vi "Main.vi"() -> ()   [LabVIEW 2018]
uses:
  Data Def/Com Port.ctl
  Data Def/Device.ctl
  <userlib>/_MGI/Timing/MGI Wait/MGI Wait (U32).vi
panel:
  in  "KFM Disconnect PLZ":bool
  in  "KFM Connect PLZ":bool
  in  "Stop Load":bool
  in  "Apply Load":bool
  out "Com Port":T1
  out "Run Count":i32
  out "Setting Tab":T2(tab)
  in  "Apply PLZ Setting":bool
  in  "Operation Mode":u16(ring) items=["Constant Current(CC)", "Constant Voltage(CV)", "Constant Power(CP)", "Constant Resistance(CR)", "Constant Current & Voltage(CCCV)", "Constant Resistance & Voltage(CRCV)"]
  out "Error":errorcluster
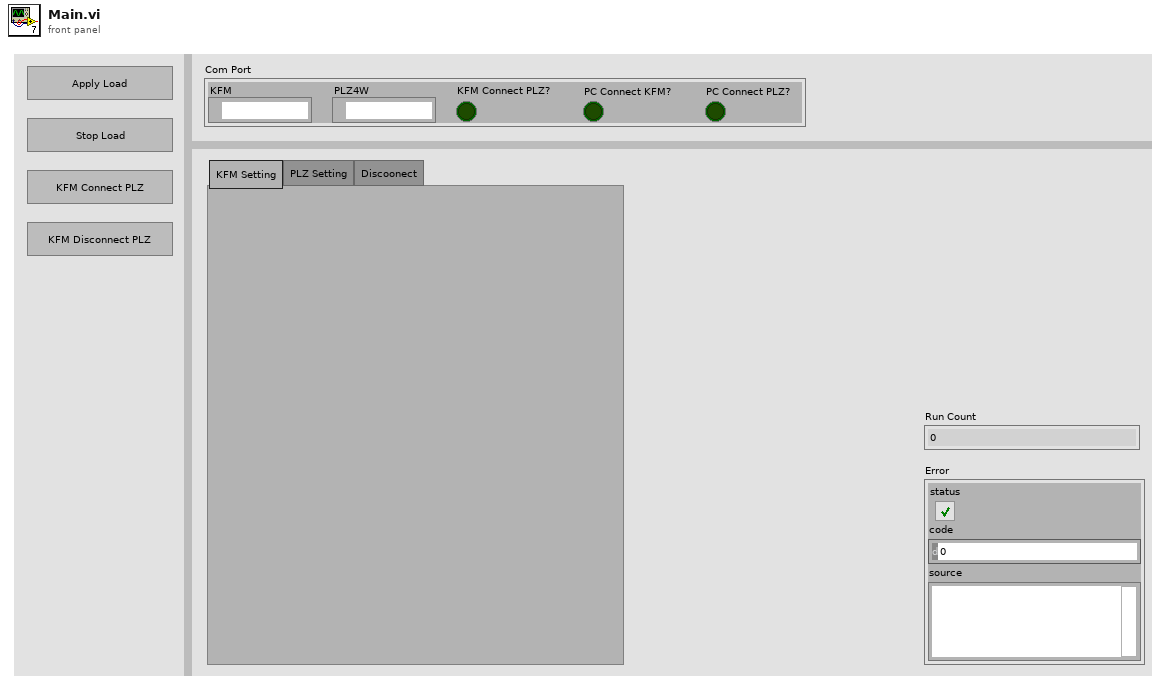
[diagram p1: front panel]
types:
  T1 = typedef "Com Port.ctl" = cluster{"KFM":refnum<visa-resource-name>, "PLZ4W":refnum<visa-resource-name>, "KFM Connect PLZ?":bool, "PC Connect KFM?":bool, "PC Connect PLZ?":bool}
  T2 = enum32{"KFM Setting", "PLZ Setting", "Discoonect"}
  T3 = typedef "Device.ctl" = enum16{"KFM", "PLZ"}
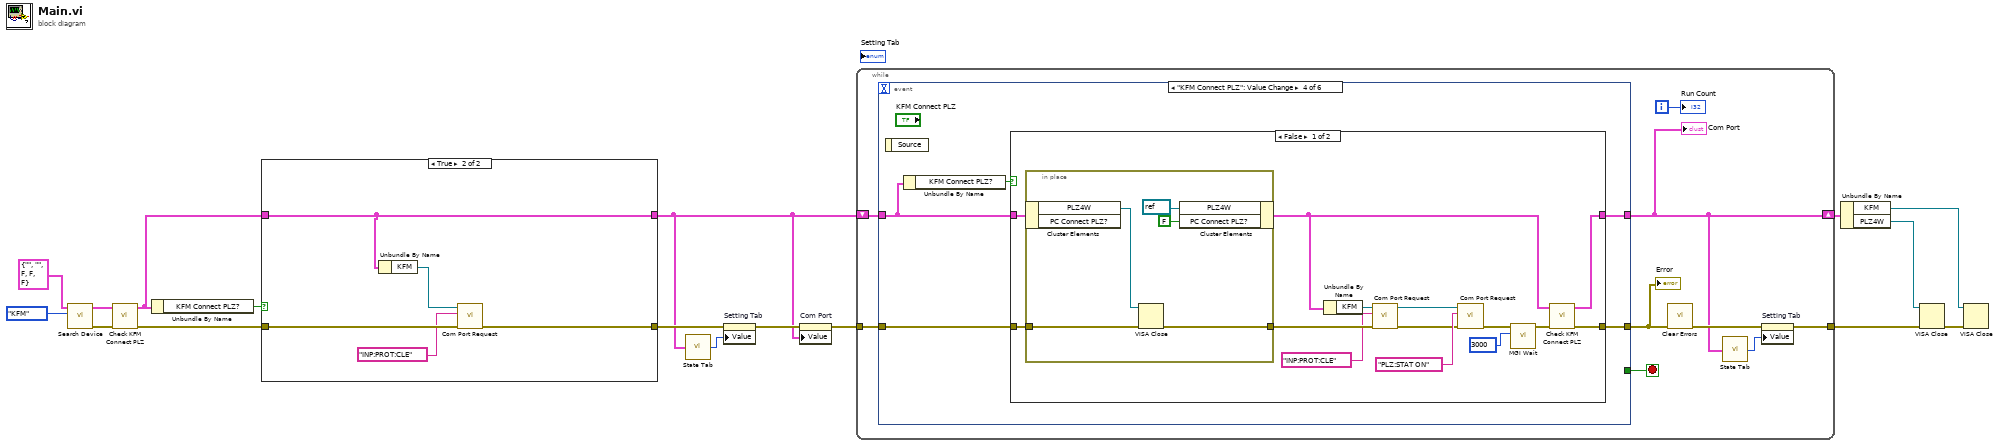
[diagram p0: block diagram]
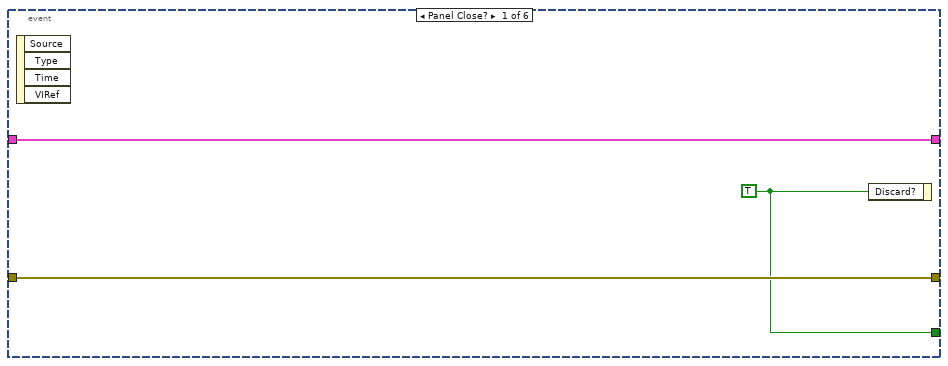
[diagram p2: hidden frame]
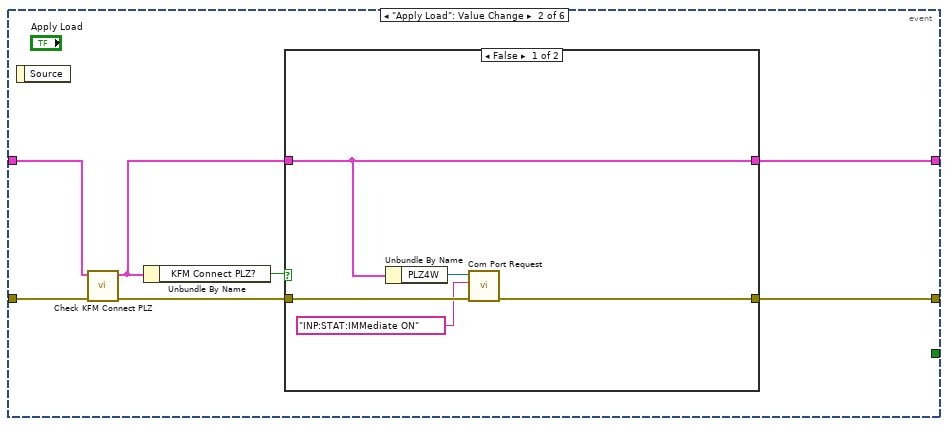
[diagram p3: hidden frame]
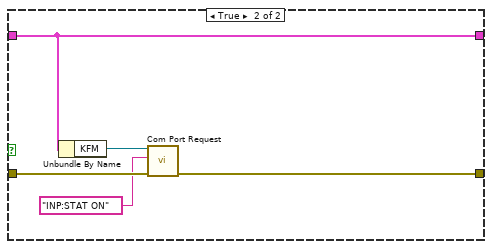
[diagram p4: hidden frame]
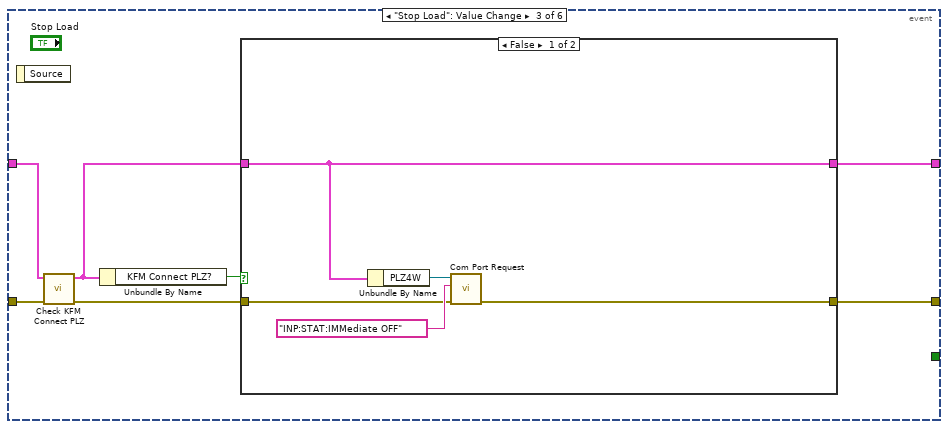
[diagram p5: hidden frame]
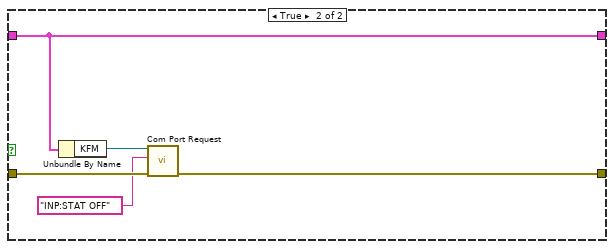
[diagram p6: hidden frame]
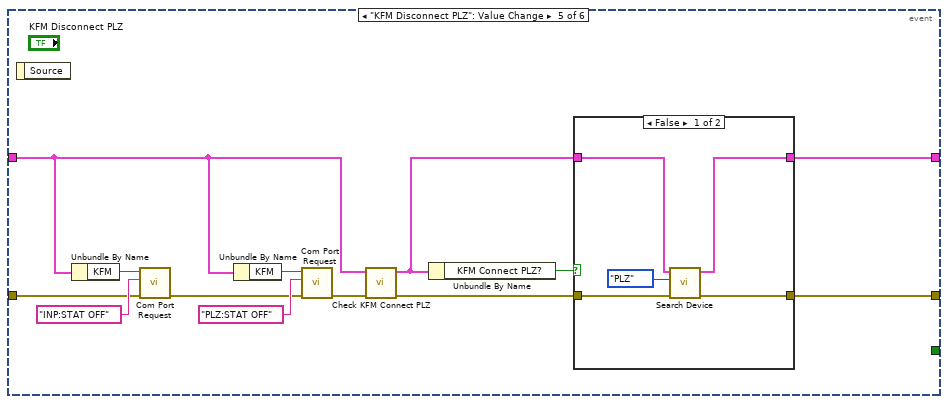
[diagram p8: hidden frame]
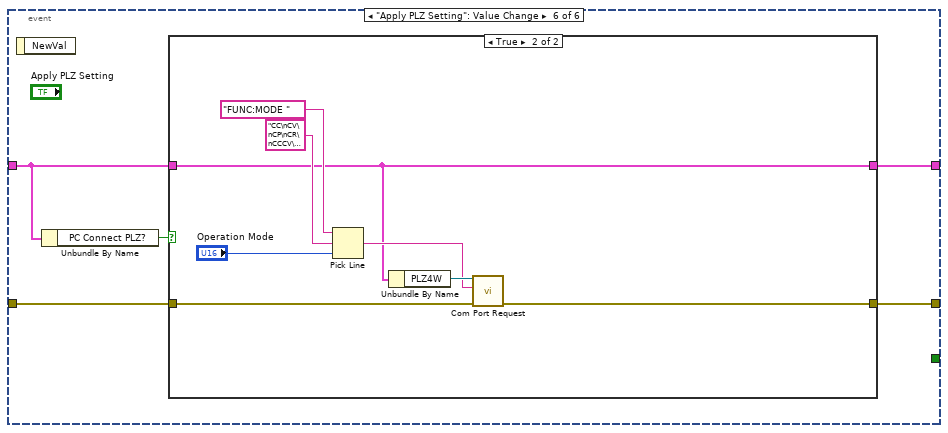
[diagram p10: hidden frame]
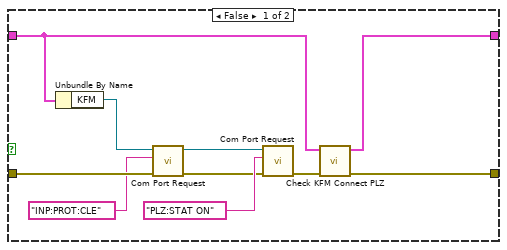
[diagram p12: hidden frame]
diagram:
  n1 = call "Search Device.vi"("Device"=Device."KFM", "Com Port In"=T1 {"KFM"="", "PLZ4W"="", "KFM Connect PLZ?"=FALSE, "PC Connect KFM?"=FALSE, "PC Connect PLZ?"=FALSE} ("Com Port")) -> ("error out"=w11:errorcluster, "Com Port Out"=w10:T1)  [unwired: 8 in]
  n2 = call "Check KFM Connect PLZ.vi"("error in"=w11, "Com Port In"=w10) -> ("error out"=w13:errorcluster, "Com Port Out"=w6:T1)  [unwired: 8 in]
  n3 = Unbundle By Name(w6) -> ("KFM Connect PLZ?"=w7:bool)
  n4 = case shown="True" w7 {
    tunnel: w13 -> [w19 w31]
    tunnel: w6 -> [w25 w29]
    tunnel: [w23 w29] -> w2
    tunnel: [w24 w28] -> w5
    frame False {
      n5 = Unbundle By Name(w25) -> ("KFM"=w21:refnum<visa-resource-name>)
      n6 = call "Com Port Request.vi"("error in"=w19, "Command"="INP:PROT:CLE", "Com Port In"=w21) -> ("error out"=w22:errorcluster, "Com Port Out"=w20:refnum<visa-resource-name>)  [unwired: 6 in, 1 out]
      n7 = call "Com Port Request.vi"("error in"=w22, "Command"="PLZ:STAT ON", "Com Port In"=w20) -> ("error out"=w26:errorcluster)  [unwired: 6 in, 2 out]
      n8 = call "Check KFM Connect PLZ.vi"("error in"=w26, "Com Port In"=w25) -> ("error out"=w24:errorcluster, "Com Port Out"=w23:T1)  [unwired: 8 in]
    }
    frame True {
      n9 = Unbundle By Name(w29) -> ("KFM"=w32:refnum<visa-resource-name>)
      n10 = call "Com Port Request.vi"("error in"=w31, "Command"="INP:PROT:CLE", "Com Port In"=w32) -> ("error out"=w28:errorcluster)  [unwired: 6 in, 2 out]
    }
  }
  n11 = call "State Tab.vi"("Com Port"=w2) -> ("Setting Tab"=w4:T2)
  n12 = property on="Setting Tab" class="TabCtl (strict)"(error in=w5, "Value"=w4) -> (error out=w3:errorcluster)  [unwired: 1 in, 1 out]
  n13 = property on="Com Port" class="Clust (strict)"(error in=w3, "Value"=w2) -> (error out=w1:errorcluster)  [unwired: 1 in, 1 out]
  n14 = while {
    tunnel: w1 -> [w40]
    shift-right: [w33] -> w14
    shift-left: w2 -> [w41]
    tunnel: [w34] -> w12
    i -> [w37]
    stop <- w39 stop-if-true
    n15 = event shown="[3] \"KFM Connect PLZ\": Value Change" {
      selector: _ -> [_ _ _ _ _ _]
      dyn-events: _ -> [_ _ _ _ _ _]
      timeout: _ -> [_ _ _ _ _ _]
      tunnel: w41 -> [w44 w47 w66 w80 w105 w128]
      tunnel: w40 -> [w43 w48 w68 w83 w107 w127]
      tunnel: [w44 w46 w64 w82 w113 w125] -> w33
      tunnel: [w43 w45 w65 w81 w114 w126] -> w38
      tunnel: [w42 _ _ _ _ _] -> w39
      event Panel Close? {
        w42 = TRUE ("Discard?")
        n16 = event-data() -> ()  [unwired: 1 in, 4 out]
        n17 = event-data("Discard?"=w42) -> ()  [unwired: 1 in, 1 out]
      }
      event "Apply Load": Value Change {
        n18 = event-data() -> ()  [unwired: 1 in, 1 out]
        n19 = call "Check KFM Connect PLZ.vi"("error in"=w48, "Com Port In"=w47) -> ("error out"=w51:errorcluster, "Com Port Out"=w50:T1)  [unwired: 8 in]
        n20 = Unbundle By Name(w50) -> ("KFM Connect PLZ?"=w49:bool)
        n21 = case shown="False" w49 {
          tunnel: w51 -> [w56 w61]
          tunnel: w50 -> [w52 w58]
          tunnel: [w53 w59] -> w45
          tunnel: [w52 w58] -> w46
          frame False {
            n22 = Unbundle By Name(w52) -> ("PLZ4W"=w55:refnum<visa-resource-name>)
            n23 = call "Com Port Request.vi"("error in"=w56, "Command"="INP:STAT:IMMediate ON", "Com Port In"=w55) -> ("error out"=w53:errorcluster)  [unwired: 6 in, 2 out]
          }
          frame True {
            n24 = Unbundle By Name(w58) -> ("KFM"=w60:refnum<visa-resource-name>)
            n25 = call "Com Port Request.vi"("error in"=w61, "Command"="INP:STAT ON", "Com Port In"=w60) -> ("error out"=w59:errorcluster)  [unwired: 6 in, 2 out]
          }
        }
      }
      event "Stop Load": Value Change {
        n26 = event-data() -> ()  [unwired: 1 in, 1 out]
        n27 = call "Check KFM Connect PLZ.vi"("error in"=w68, "Com Port In"=w66) -> ("error out"=w67:errorcluster, "Com Port Out"=w63:T1)  [unwired: 8 in]
        n28 = Unbundle By Name(w63) -> ("KFM Connect PLZ?"=w62:bool)
        n29 = case shown="False" w62 {
          tunnel: w67 -> [w71 w78]
          tunnel: w63 -> [w70 w75]
          tunnel: [w69 w76] -> w65
          tunnel: [w70 w75] -> w64
          frame False {
            n30 = Unbundle By Name(w70) -> ("PLZ4W"=w73:refnum<visa-resource-name>)
            n31 = call "Com Port Request.vi"("error in"=w71, "Command"="INP:STAT:IMMediate OFF", "Com Port In"=w73) -> ("error out"=w69:errorcluster)  [unwired: 6 in, 2 out]
          }
          frame True {
            n32 = Unbundle By Name(w75) -> ("KFM"=w77:refnum<visa-resource-name>)
            n33 = call "Com Port Request.vi"("error in"=w78, "Command"="INP:STAT OFF", "Com Port In"=w77) -> ("error out"=w76:errorcluster)  [unwired: 6 in, 2 out]
          }
        }
      }
      event "KFM Connect PLZ": Value Change {
        n34 = event-data() -> ()  [unwired: 1 in, 1 out]
        n35 = Unbundle By Name(w80) -> ("KFM Connect PLZ?"=w79:bool)
        n36 = case shown="False" w79 {
          tunnel: w83 -> [w97 w104]
          tunnel: [w94 w103] -> w82
          tunnel: [w93 w104] -> w81
          tunnel: w80 -> [w84 w103]
          frame False {
            n37 = in-place {
              in-place-border: w97 -> [w102]
              in-place-border: [w99] -> w92
              n38 = in-place-cluster #1(w84) -> ("PLZ4W"=w101:refnum<visa-resource-name>)  [unwired: 1 out]
              n39 = VISA Close(VISA resource name=w101, error in (no error)=w102) -> (error out=w99:errorcluster)
              n40 = in-place-cluster #1("PLZ4W"=refnum<visa-resource-name> refnum, "PC Connect PLZ?"=FALSE) -> (w95:T1)
            }
            n41 = Unbundle By Name(w95) -> ("KFM"=w89:refnum<visa-resource-name>)
            n42 = call "Com Port Request.vi"("error in"=w92, "Command"="INP:PROT:CLE", "Com Port In"=w89) -> ("error out"=w91:errorcluster, "Com Port Out"=w90:refnum<visa-resource-name>)  [unwired: 6 in, 1 out]
            n43 = call "Com Port Request.vi"("error in"=w91, "Command"="PLZ:STAT ON", "Com Port In"=w90) -> ("error out"=w87:errorcluster)  [unwired: 6 in, 2 out]
            n44 = call-poly <userlib>:"MGI Wait.vi"("ms"=u32 3000, "Error In"=w87) -> ("Error Out"=w86:errorcluster)  [unwired: 5 in]
            n45 = call "Check KFM Connect PLZ.vi"("error in"=w86, "Com Port In"=w95) -> ("error out"=w93:errorcluster, "Com Port Out"=w94:T1)  [unwired: 8 in]
          }
          frame True {
          }
        }
      }
      event "KFM Disconnect PLZ": Value Change {
        n46 = event-data() -> ()  [unwired: 1 in, 1 out]
        n47 = Unbundle By Name(w105) -> ("KFM"=w108:refnum<visa-resource-name>)
        n48 = call "Com Port Request.vi"("error in"=w107, "Command"="INP:STAT OFF", "Com Port In"=w108) -> ("error out"=w106:errorcluster)  [unwired: 6 in, 2 out]
        n49 = Unbundle By Name(w105) -> ("KFM"=w117:refnum<visa-resource-name>)
        n50 = call "Com Port Request.vi"("error in"=w106, "Command"="PLZ:STAT OFF", "Com Port In"=w117) -> ("error out"=w116:errorcluster)  [unwired: 6 in, 2 out]
        n51 = call "Check KFM Connect PLZ.vi"("error in"=w116, "Com Port In"=w105) -> ("error out"=w112:errorcluster, "Com Port Out"=w111:T1)  [unwired: 8 in]
        n52 = Unbundle By Name(w111) -> ("KFM Connect PLZ?"=w110:bool)
        n53 = case shown="False" w110 {
          tunnel: [w122 w123] -> w114
          tunnel: [w120 w124] -> w113
          tunnel: w112 -> [w119 w123]
          tunnel: w111 -> [w118 w124]
          frame False {
            n54 = call "Search Device.vi"("error in"=w119, "Device"=Device."PLZ", "Com Port In"=w118) -> ("error out"=w122:errorcluster, "Com Port Out"=w120:T1)  [unwired: 7 in]
          }
          frame True {
          }
        }
      }
      event "Apply PLZ Setting": Value Change {
        n55 = event-data() -> ()  [unwired: 1 in, 1 out]
        n56 = Unbundle By Name(w128) -> ("PC Connect PLZ?"=w129:bool)
        n57 = case shown="True" w129 {
          tunnel: w128 -> [w130 w132]
          tunnel: w127 -> [w131 w136]
          tunnel: [w131 w133] -> w126
          tunnel: [w130 w132] -> w125
          frame False {
          }
          frame True {
            n58 = Pick Line(string ("")="FUNC:MODE ", multi-line string="CC\nCV\nCP\nCR\nCCCV\nCRCV", line index="Operation Mode") -> (output string=w134:string)
            n59 = Unbundle By Name(w132) -> ("PLZ4W"=w135:refnum<visa-resource-name>)
            n60 = call "Com Port Request.vi"("error in"=w136, "Command"=w134, "Com Port In"=w135) -> ("error out"=w133:errorcluster)  [unwired: 6 in, 2 out]
          }
        }
      }
    }
    "Error" <- w38
    "Com Port" <- w33
    n61 = call <vilib>:"Clear Errors.vi"("error in (no error)"=w38) -> ("error out"=w35:errorcluster)  [unwired: 5 in, 1 out]
    n62 = call "State Tab.vi"("Com Port"=w33) -> ("Setting Tab"=w36:T2)
    n63 = property on="Setting Tab" class="TabCtl (strict)"(error in=w35, "Value"=w36) -> (error out=w34:errorcluster)  [unwired: 1 in, 1 out]
    "Run Count" <- w37
  }
  n64 = Unbundle By Name(w14) -> ("KFM"=w15:refnum<visa-resource-name>, "PLZ4W"=w17:refnum<visa-resource-name>)
  n65 = VISA Close(VISA resource name=w17, error in (no error)=w12) -> (error out=w16:errorcluster)
  n66 = VISA Close(VISA resource name=w15, error in (no error)=w16) -> ()  [unwired: 1 out]
